vi "AD_Conv.vi"(6 "HEAD":T1={"File"=[refnum], "Idx"=[], "dT"=0.5, "Hd"=4096, "Rd"=14, "Start"=[timestamp(3519879471 s since 1904-01-01)], "Trig"=[timestamp(3519879472 s since 1904-01-01)], "Stop"=[timestamp(3519940623 s since 1904-01-01)], "FirstPos"=[], "Count"=[120609], "Color"=[27836, 4765252, 11010216, 14712848], "Label"=["CH1", "CH2", "CH3", "CH4"], "INP"=["CH1", "CH2", "CH3", "CH4"], "H"=[5.0, 5.0, 5.0, 5.0], "L"=[-5.0, -5.0, -5.0, -5.0], "Fmt"=["%.;%+0.3f V", "%.;%+0.3f V", "%.;%+0.3f V", "%.;%+0.3f V"], "Unit"=["", "", "", ""], "SEL"=[0, 1, 2, 3], "Byte"=[-2, -2, -2, -2], "Pos"=[], "Bit"=[], "Flg"=[], "Gain"=[], "Offset"=[0.01, 0.01, 0.01, 0.01], "CH"=[0, 0, 0, 0], "Opt"={"Mode"=0, "TUNIT"=enum."CELS"}, "TYPE"=enum."GBD", "Comp"=[], "Temp"=[]} {"FirstPos" format="%<%x %.3X>T"; "Stop" format="%<%x %.3X>T"; "Trig" format="%<%x %.3X>T"; "Start" format="%<%x %.3X>T"}, 8 "No":i32, 11 "ACK":i32) -> (3 "Data":dbl)   [LabVIEW 2017]
uses:
  Amp_Param.ctl
  Driver/TempConv.dll
panel:
  in  "Temp":bool
  # "ALL"
  # "GBD"
  # "CSV"
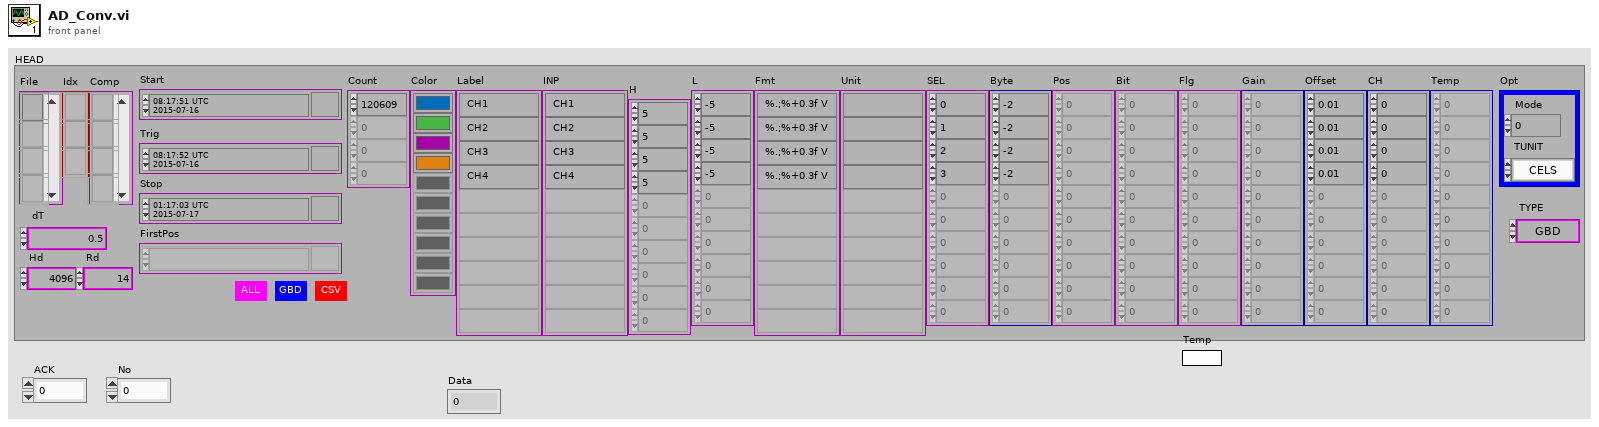
[diagram p1: front panel]
types:
  T1 = typedef "Amp_Param.ctl" = cluster{"File":refnum<file>[], "Idx":refnum<file>[], "dT":dbl, "Hd":i32, "Rd":i32, "Start":timestamp[], "Trig":timestamp[], "Stop":timestamp[], "FirstPos":timestamp[], "Count":i64[], "Color":u32[], "Label":string[], "INP":string[], "H":dbl[], "L":dbl[], "Fmt":string[], "Unit":string[], "SEL":i32[], "Byte":i32[], "Pos":i32[], "Bit":i32[], "Flg":i32[], "Gain":dbl[], "Offset":dbl[], "CH":i32[], "Opt":cluster{"Mode":i32, "TUNIT":enum16{"CELS", "FAHR"}}, "TYPE":enum16{"GBD", "CSV"}, "Comp":refnum<file>[], "Temp":i32[]}
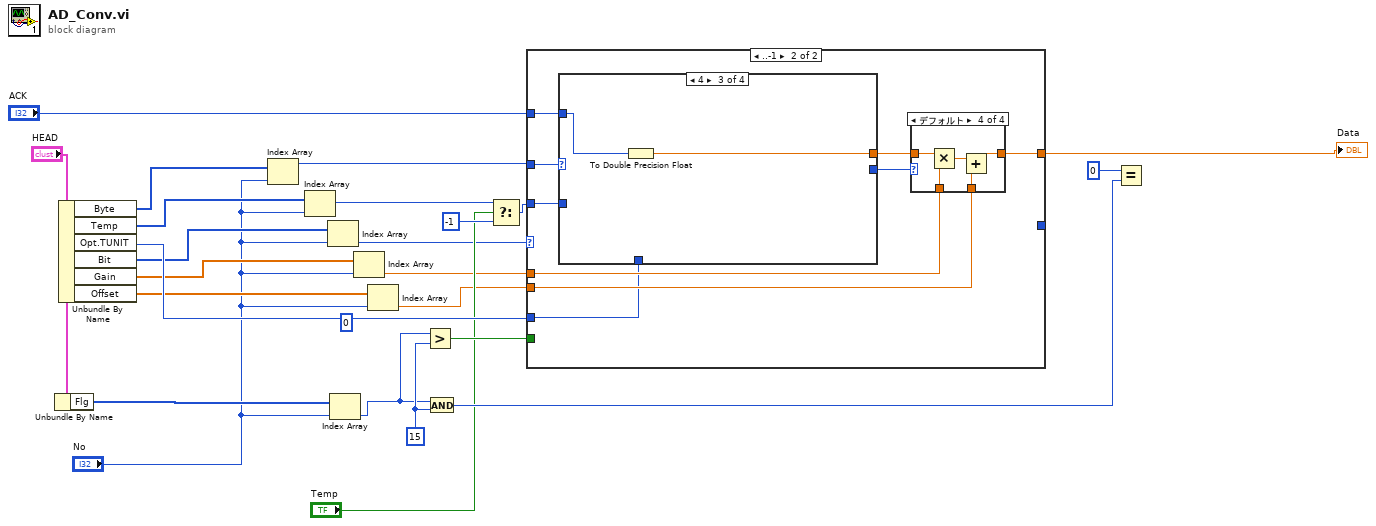
[diagram p0: block diagram]
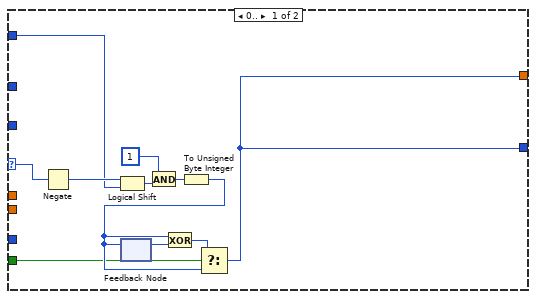
[diagram p2: hidden frame]
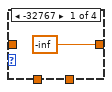
[diagram p3: hidden frame]
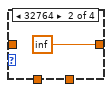
[diagram p4: hidden frame]
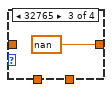
[diagram p5: hidden frame]
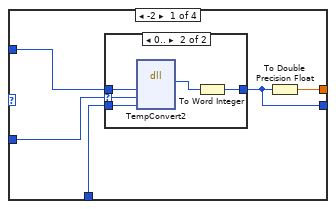
[diagram p6: hidden frame]
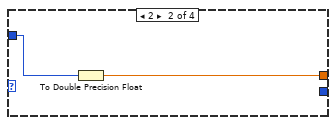
[diagram p8: hidden frame]
diagram:
  (unwired) u8 0
  w19 = 15 ("x")
  n1 = Unbundle By Name("HEAD") -> ("Flg"=w4:i32[])
  n2 = Unbundle By Name("HEAD") -> ("Byte"=w15:i32[], "Temp"=w13:i32[], "Opt.TUNIT"=w12:enum16{"CELS", "FAHR"}, "Bit"=w10:i32[], "Gain"=w8:dbl[], "Offset"=w6:dbl[])
  n3 = Index Array(array=w15, index="No") -> (element=w14:i32)
  n4 = Index Array(array=w13, index="No") -> (element=w21:i32)
  n5 = Index Array(array=w10, index="No") -> (element=w9:i32)
  n6 = Index Array(array=w4, index="No") -> (element=w2:i32)
  n7 = Index Array(array=w8, index="No") -> (element=w7:dbl)
  n8 = Index Array(array=w6, index="No") -> (element=w5:dbl)
  n9 = Greater?(x=w2, y=w19) -> (0:w20:bool)
  n10 = And(x=w2, y=w19) -> (x .and. y?=w18:i32)
  n11 = Select(t=w21, s="Temp", f=-1) -> (s? t:f=w22:i32)
  n12 = case shown="..-1" w9 {
    selector: w9 -> [w31 _]
    tunnel: w14 -> [_ w44]
    tunnel: w7 -> [_ w41]
    tunnel: w5 -> [_ w40]
    tunnel: [w26 w39] -> w1
    tunnel: [w26 _] -> _
    tunnel: w20 -> [w28 _]
    tunnel: w22 -> [_ w38]
    tunnel: w12 -> [_ w37]
    tunnel: "ACK" -> [w25 w36]
    frame 0.. {
      n13 = Negate(x=w31) -> (-x=w35:i32)
      n14 = Logical Shift(y=w35, x=w25) -> (x << y=w33:i32)
      n15 = feedback #1() -> (w30:u8)  [unwired: 1 in]
      n16 = And(x=i16 1 ("y"), y=w33) -> (x .and. y?=w34:i32)
      n17 = To Unsigned Byte Integer(number=w34) -> (unsigned 8bit integer=w29:u8)
      n18 = feedback-in #1(w29) -> ()
      n19 = Exclusive Or(1:w30, 2:w29) -> (0:w27:u8)
      n20 = Select(t=w27, s=w28, f=w29) -> (s? t:f=w26:u8)
    }
    frame ..-1 {
      n21 = case shown="4" w44 {
        tunnel: [w57 w65 w67 _] -> w43
        tunnel: [w56 _ _ _] -> w42
        tunnel: w38 -> [w55 _ _ _]
        tunnel: w37 -> [w54 _ _ _]
        tunnel: w36 -> [w53 w64 w66 _]
        frame -2 {
          n22 = case shown="0.." w55 {
            selector: w55 -> [_ w63]
            tunnel: w53 -> [w58 w60]
            tunnel: w54 -> [_ w62]
            tunnel: [w58 w59] -> w56
            frame ..-1 {
            }
            frame 0.. {
              n23 = dll-call lib="D:/src/LabVIEW/GL860/JP/LabView VI/Driver/TempConv.dll" fn="TempConvert2"("AdData"=w60, "TcCode"=w63, "TempUnit"=w62) -> ("return type"=w61:i32)  [unwired: 6 in, 2 out]
              n24 = To Word Integer(number=w61) -> (16bit integer=w59:i16)
            }
          }
          n25 = To Double Precision Float(number=w56) -> (double precision float=w57:dbl)
        }
        frame 2 {
          n26 = To Double Precision Float(number=w64) -> (double precision float=w65:dbl)
        }
        frame 4 {
          n27 = To Double Precision Float(number=w66) -> (double precision float=w67:dbl)
        }
        frame Default {
        }
      }
      n28 = case shown="デフォルト" w42 {
        tunnel: w43 -> [_ _ _ w51]
        tunnel: [-inf ("Numeric") inf ("Numeric") nan ("Numeric") w50] -> w39
        tunnel: w40 -> [_ _ _ w49]
        tunnel: w41 -> [_ _ _ w48]
        frame -32767 {
        }
        frame 32764 {
        }
        frame 32765 {
        }
        frame Default {
          n29 = Multiply(x=w51, y=w48) -> (x*y=w52:dbl)
          n30 = Add(x=w52, y=w49) -> (x+y=w50:dbl)
        }
      }
    }
  }
  "Data" <- w1
  n31 = Equal?(x=0, y=w18) -> ()  [unwired: 1 out]
